vi "Write to Message Log.vi"(8 "error in (no error)":errorcluster, 11 "Message":string) -> (0 "error out":errorcluster)   [LabVIEW 2015, in "UI Handler.lvclass"]
uses:
  UI Handler.lvclass
  UI Handler.lvclass/UI Handler.ctl
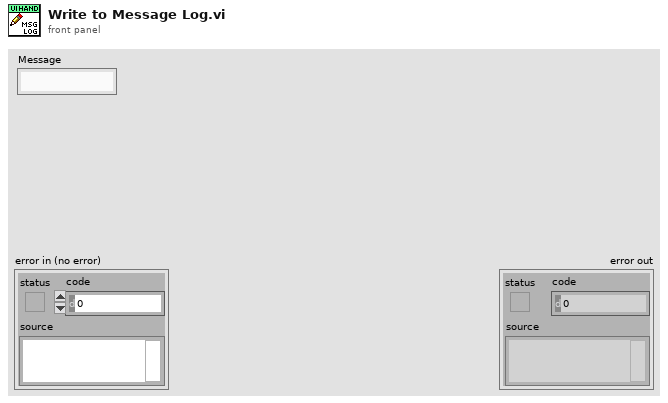
[diagram p1: front panel]
types:
  T1 = typedef "UI Handler.lvclass/Session Handle.ctl" = refnum<data-value>
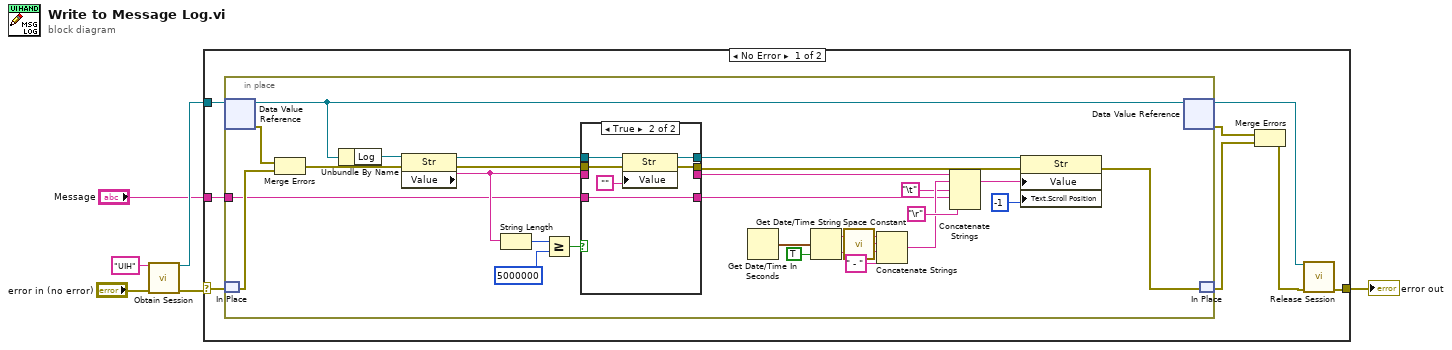
[diagram p0: block diagram]
diagram:
  n1 = call "Obtain Session.vi"("Session  Name ()"="UIH", "error in (no error)"="error in (no error)") -> ("Session Handle"=w2:T1, "error out"=w3:errorcluster)  [unwired: 12 in]
  n2 = case shown="No Error" w3 {
    selector: w3 -> [w11 w53]
    tunnel: w2 -> [w14 _]
    tunnel: [w7 w53] -> w5
    tunnel: "Message" -> [w10 _]
    frame No Error {
      n3 = in-place {
        in-place-border: w10 -> [w17]
        n4 = in-place-dvr #1(w14) -> (w42:refnum<class "UI Handler.lvclass">, w29:errorcluster)
        n5 = in-place-match #2(w11) -> (w28:errorcluster)
        n6 = Merge Errors(w29, w28) -> (w27:errorcluster)
        n7 = Unbundle By Name(w42) -> ("Log"=w30:refnum<vi>)
        n8 = property class="Str"(reference=w30, error in=w27) -> (reference out=w22:refnum<vi>, error out=w21:errorcluster, "Value"=w20:string)
        n9 = String Length(string=w20) -> (length=w25:i32)
        n10 = Greater Or Equal?(x=w25, y=5000000) -> (x >= y?=w23:bool)
        n11 = case shown="True" w23 {
          tunnel: w22 -> [w46 w52]
          tunnel: w21 -> [w45 w51]
          tunnel: w20 -> [w43 _]
          tunnel: [w46 w50] -> w19
          tunnel: [w45 w49] -> w18
          tunnel: [w44 w47] -> w16
          tunnel: w17 -> [w44 w47]
          tunnel: [w43 _] -> w15
          frame False {
          }
          frame True {
            n12 = property class="Str"(reference=w52, error in=w51, "Value"="") -> (reference out=w50:refnum<vi>, error out=w49:errorcluster)
          }
        }
        n13 = Get Date/Time In Seconds() -> (seconds since 1Jan1904=w38:timestamp)
        n14 = Get Date/Time String(seconds (now)=w38, want seconds? (F)=TRUE) -> (date string=w36:string, time string=w35:string)  [unwired: 1 in]
        n15 = call <vilib>:"Space Constant.vi"() -> ("String"=w32:string)
        n16 = Concatenate Strings(w36, w32, w35, " - " ("string")) -> (w34:string)
        n17 = Concatenate Strings(w15, w34, "\t", w16, "\r") -> (w40:string)
        n18 = property class="Str"(reference=w19, error in=w18, "Value"=w40, "Text.Scroll Position"=-1) -> (error out=w26:errorcluster)  [unwired: 1 out]
        n19 = in-place-dvr #1(w42) -> (w8:T1, w12:errorcluster)
        n20 = in-place-match #2(w26) -> (w13:errorcluster)
      }
      n21 = Merge Errors(w12, w13) -> (w9:errorcluster)
      n22 = call "Release Session.vi"("Session Handle"=w8, "error in (no error)"=w9) -> ("error out"=w7:errorcluster)  [unwired: 13 in]
    }
    frame Error {
    }
  }
  "error out" <- w5
